vi "WPI_UtilitiesClearTestMode.vi"(11 "Tree Refnum":refnum<vi>) -> ()   [LabVIEW 2017]
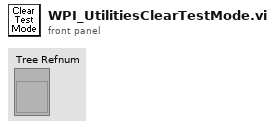
[diagram p1: front panel]
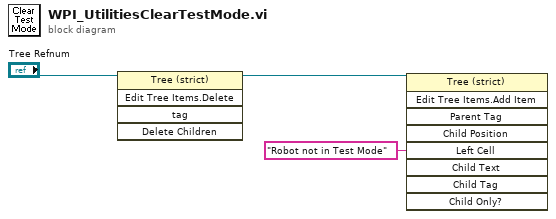
[diagram p0: block diagram]
diagram:
  n1 = invoke class="Tree (strict)" method="Edit Tree Items.Delete"(reference="Tree Refnum") -> (reference out=w2:refnum<vi>)  [unwired: 4 in, 4 out]
  n2 = invoke class="Tree (strict)" method="Edit Tree Items.Add Item"(reference=w2, "Left Cell"="Robot not in Test Mode" ("Left Cell String")) -> ()  [unwired: 7 in, 9 out]
